vi "Noise_filtering.vi"(6 "Array 3":sgl[](array[numeric]), 7 "Array in":sgl[](array[numeric]), 9 "Array 4":sgl[](array[numeric]), 10 "Array 5":sgl[](array[numeric]), 11 "Array 6":sgl[](array[numeric])) -> (3 "Array out":dbl[](array[numeric]))   [LabVIEW 2021]
doc: "This VI takes previous ball coordinates and returns a moving average of these coordinates"
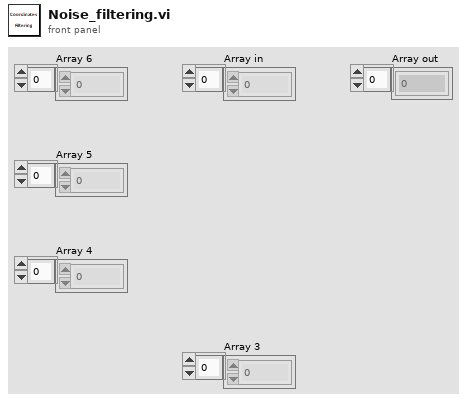
[diagram p1: front panel]
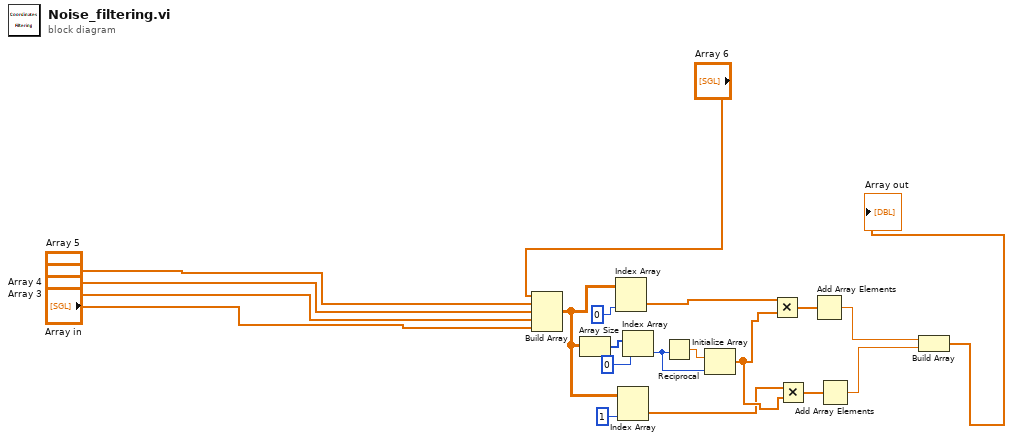
[diagram p0: block diagram]
diagram:
  n1 = Build Array("Array 6", "Array 5", "Array 4", "Array 3", "Array in") -> (w6:sgl[][])
  n2 = Array Size(array=w6) -> (size(s)=w2:i32[])
  n3 = Index Array(array=w6, index (col)=0 ("length")) -> (element=w8:sgl[])  [unwired: 1 in]
  n4 = Index Array(array=w6, index (col)=1 ("disabled index (col)")) -> (element=w11:sgl[])  [unwired: 1 in]
  n5 = Index Array(array=w2, index=0) -> (element=w4:i32)
  n6 = Reciprocal(x=w4) -> (1/x=w3:dbl)
  n7 = Initialize Array(w3, w4) -> (w12:dbl[])
  n8 = Multiply(x=w8, y=w12) -> (x*y=w9:dbl[])
  n9 = Multiply(x=w11, y=w12) -> (x*y=w10:dbl[])
  n10 = Add Array Elements(numeric array=w9) -> (sum=w13:dbl)
  n11 = Add Array Elements(numeric array=w10) -> (sum=w14:dbl)
  n12 = Build Array(w13, w14) -> (→"Array out":dbl[])
